vi "Process_Backup.vi"(8 "error in":errorcluster, 11 "RemoteControl":refnum<class "RemoteControl.lvclass">) -> (0 "error out":errorcluster, 3 "RemoteControl out":refnum<class "RemoteControl.lvclass">)   [LabVIEW 2016]
doc: "---------------------------------------------------------------\nJKI State Machine Objects™\nhttp://jki.net/state-machine-objects/\nCopyright (C) 2005-2015, JKI <info@jki.net>\nALL RIGHTS RESERVED"
uses:
  RemoteControl.lvclass
  <vilib>/JKI/JKI SMO/SMO/SMO.lvclass
  <vilib>/JKI/JKI SMO/SMO/Typedefs/Parent Call--Enum.ctl
  Typedefs/Message--Cluster.ctl
  Typedefs/PublicEvents--RemoteControl.SendMessageFromProcess.ctl
  <vilib>/JKI/JKI SMO/SMO/Typedefs/SMOState --Enum.ctl
  C:/user/patrick/hg/levylab_inst/lvsrc/SMOs/LevyLab/LevyLab.lvclass
  C:/Program Files (x86)/National Instruments/LabVIEW 2016/vi.lib/JKI/JKI SMO/SMO/SMO.lvclass
  Typedefs/RC Process Type--Enum.ctl
panel:
  in  "Debug Mode":bool=TRUE
  out "Servers":T1[](array[typedef])
  in  "timeout in ms (100)":i32=10
  out "Message from Server":T2 {"Message ID" format="%#_6f"}
  out "Name":string
  out "Message from Remote":T2 {"Message ID" format="%#_6f"}
  out "Message from Owner":T2 {"Message ID" format="%#_6f"}
  in  "stop":bool
  out "RC Process Type":T3
  # "For instructions on how to use the JKI State Machine Objects, examples and video tutorials, visit:\nhttp://jki.net/state-machine-objects/\n\nJKI State Machine Objects™\nhttp://jki.net/state-machine-objects/\nCopyright (C) 2005-2015, JKI <info@jki.net>\nALL RIGHTS RESERVED"
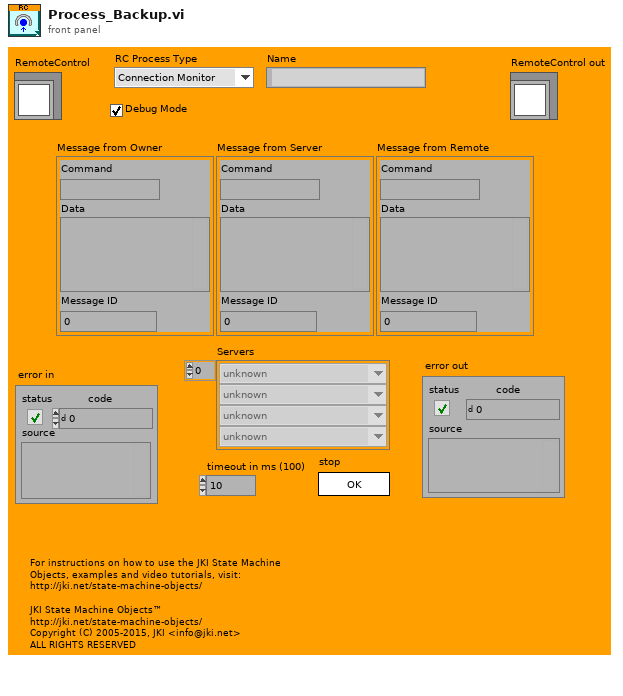
[diagram p1: front panel]
types:
  T1 = typedef "SMO.lvclass/SMOState --Enum.ctl" = enum16{"unknown", "Created", "Started", "Stopped"}
  T2 = typedef "RemoteControl.lvclass/Message--Cluster.ctl" = cluster{"Command":string, "Data":variant, "Message ID":i32}
  T3 = typedef "RemoteControl.lvclass/RC Process Type--Enum.ctl" = enum16{"Connection Monitor", "Server", "Client"}
  T4 = typedef "SMO.lvclass/Parent Call--Enum.ctl" = enum16{"Allows parent to run", "Does not request parent to run"}
  T5 = enum32{"invalid app kind", "Development System", "Run Time System", "Student Edition", "Embedded LabVIEW", "Evaluation", "Custom"}
  T6 = enum32{"Invalid", "Standard", "Closed", "Hidden", "Minimized", "Maximized"}
  T7 = enum32{"Bad", "Idle", "Run top level", "Running"}
  T8 = cluster{"Current VI Reference":refnum<vi>, "Close Panel on Exit?":bool, "error":errorcluster}
  T9 = cluster{"Core":cluster{"Current VI Reference":refnum<vi>, "Close Panel on Exit?":bool, "error":errorcluster}, "Self Reference":refnum<class "RemoteControl.lvclass">, "RC Process Type":void, "Configure":void, "Message":T2, "Servers":refnum<class "RemoteControl.lvclass">[], "Server Message":refnum<user-event>[], "Server State":refnum<user-event>[], "Server index":i32}
  T10 = typedef "SMO.lvclass/Protected Events.ctl" = cluster{"StopProcesses":refnum<user-event>, "AbortProcesses":refnum<user-event>, "Config Changed":refnum<user-event>, "Dependency":refnum<user-event>}
  T11 = typedef "RemoteControl.lvclass/PrivateEvents--Cluster.ctl" = cluster{"Configure":refnum<user-event>, "SendMessageToProcess":refnum<user-event>}
  T12 = typedef "RemoteControl.lvclass/PublicEvents--Cluster.ctl" = cluster{"SendMessageFromProcess":refnum<user-event>}
  T13 = typedef "SMO.lvclass/Public Events.ctl" = cluster{"Error":refnum<user-event>, "State":refnum<user-event>, "Reserve State":refnum<user-event>}
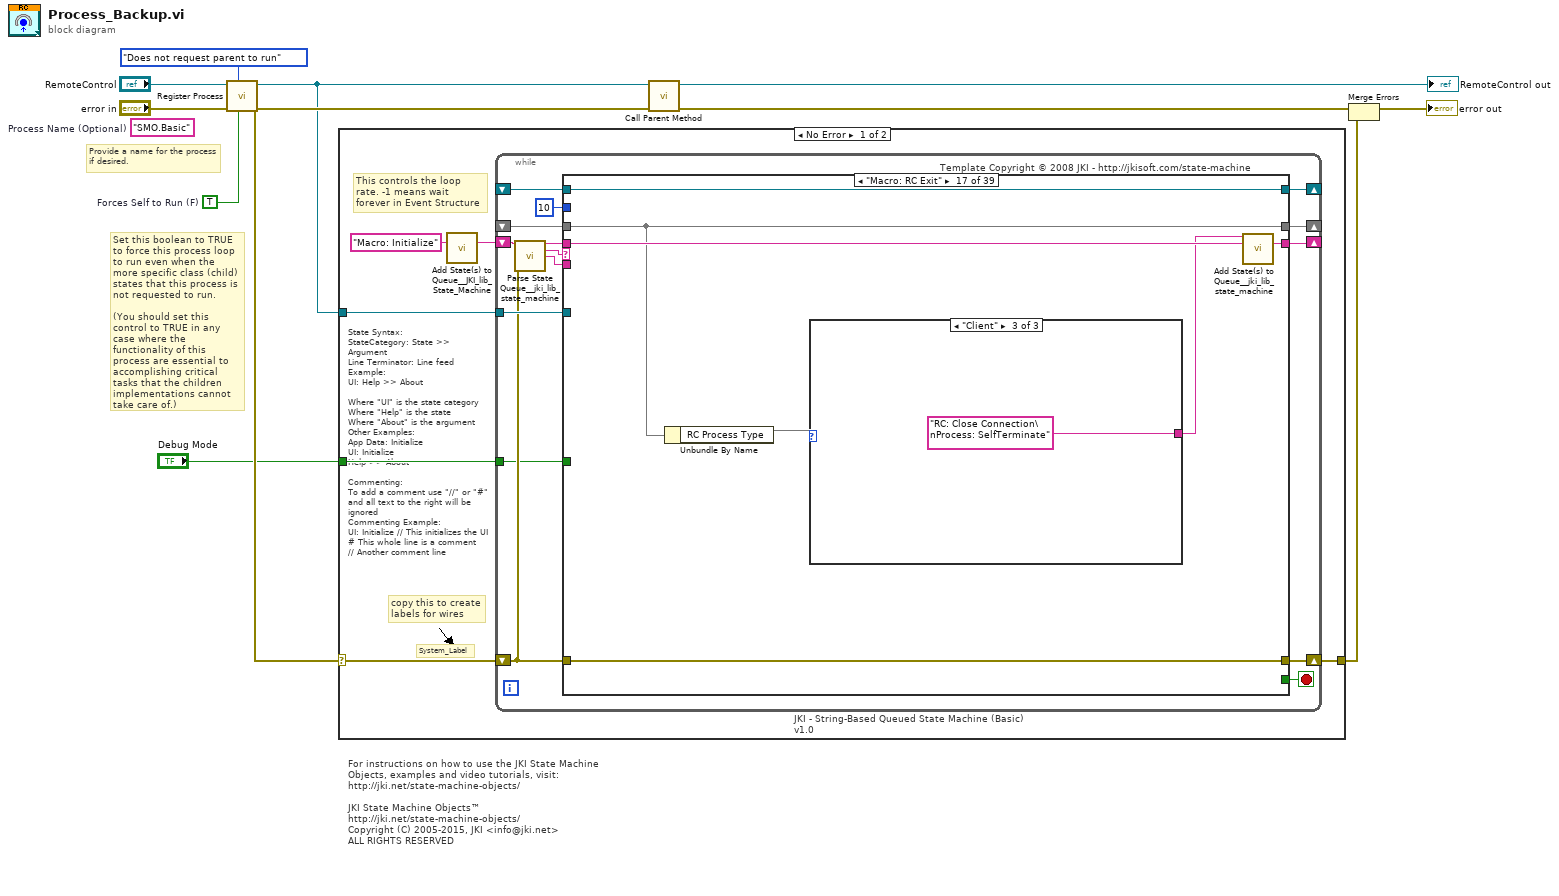
[diagram p0: block diagram]
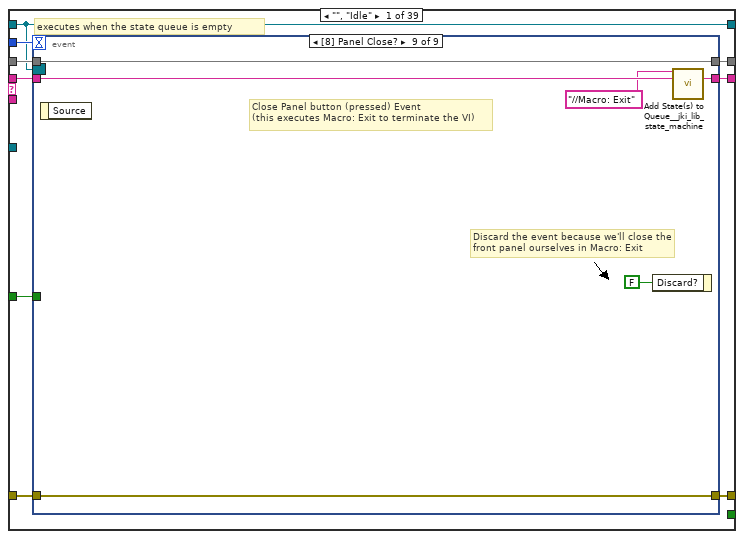
[diagram p2: hidden frame]
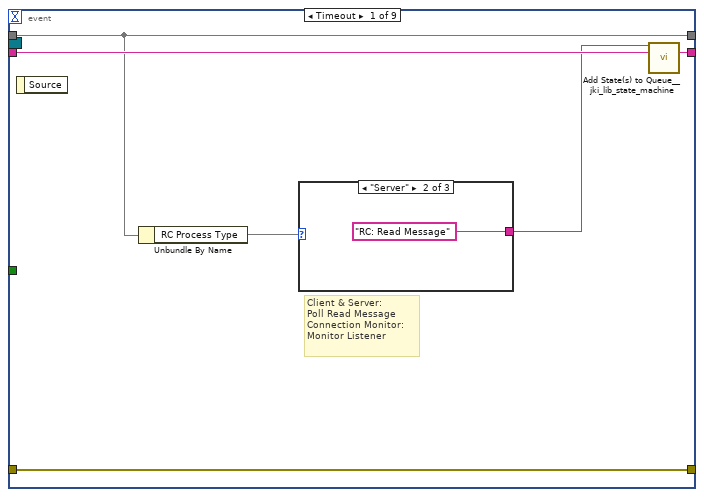
[diagram p3: hidden frame]
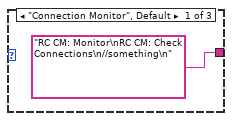
[diagram p4: hidden frame]
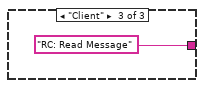
[diagram p5: hidden frame]
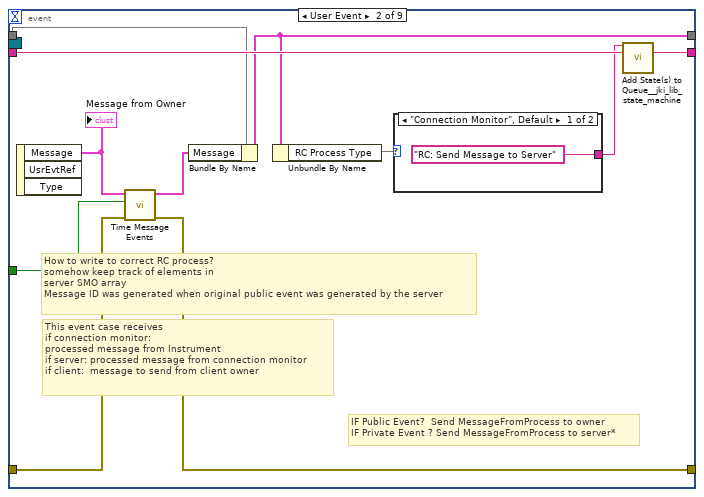
[diagram p6: hidden frame]
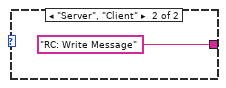
[diagram p7: hidden frame]
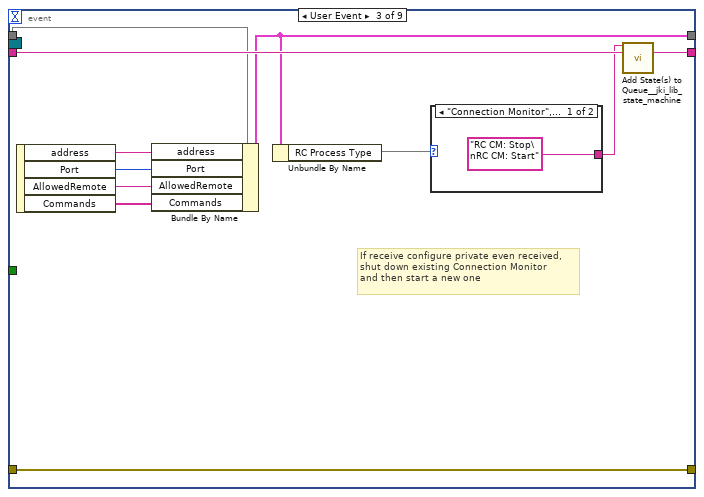
[diagram p8: hidden frame]
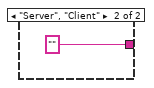
[diagram p9: hidden frame]
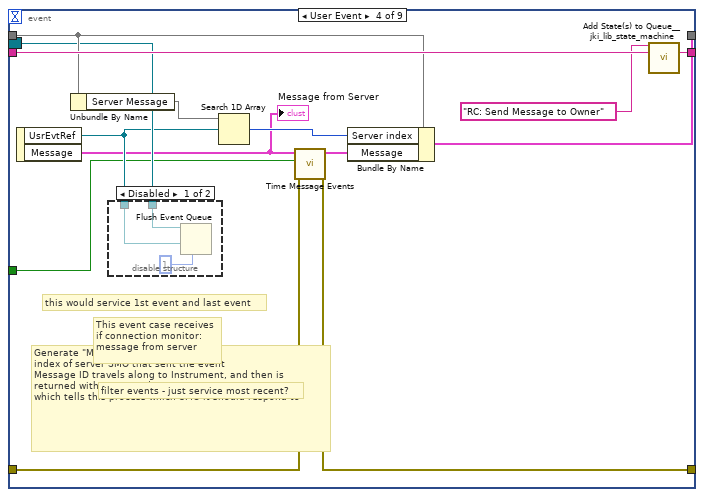
[diagram p10: hidden frame]
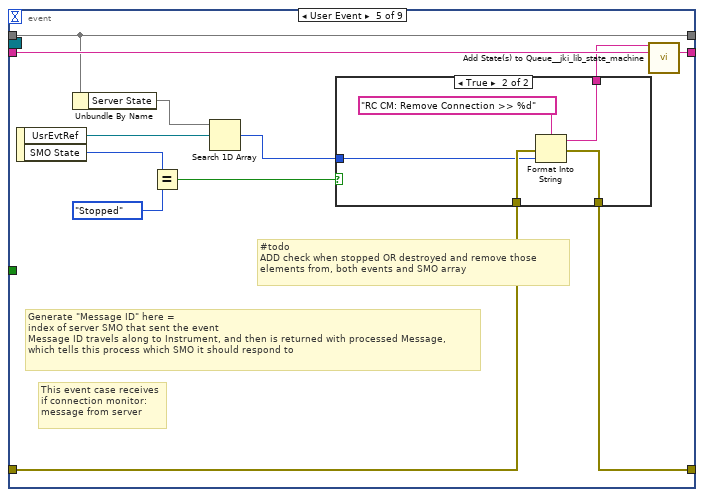
[diagram p12: hidden frame]
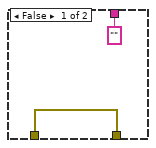
[diagram p13: hidden frame]
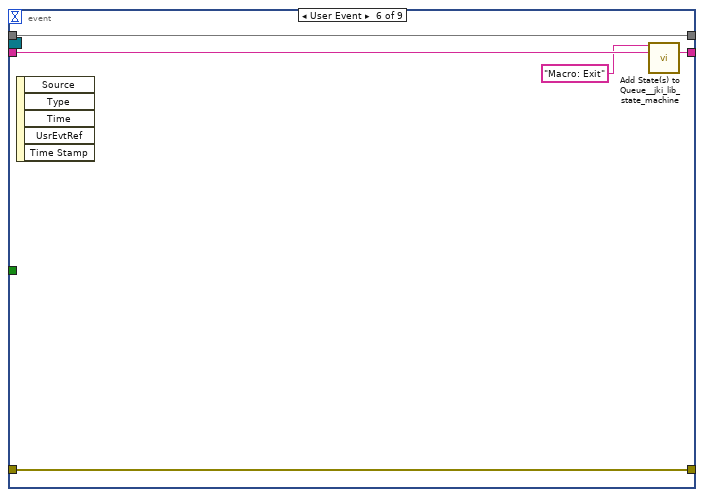
[diagram p14: hidden frame]
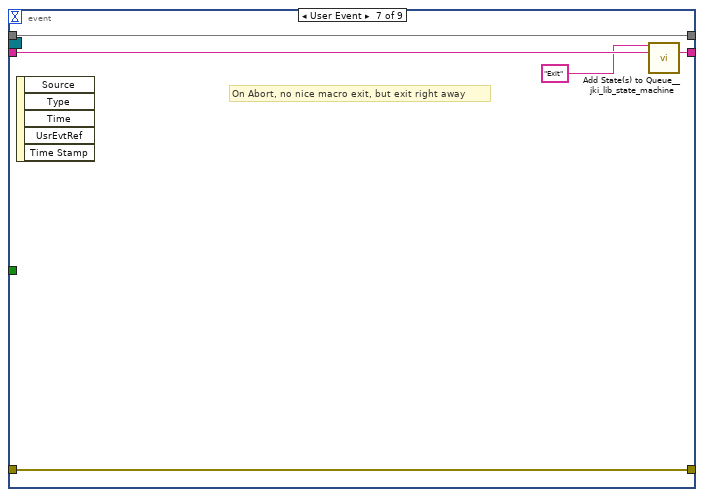
[diagram p15: hidden frame]
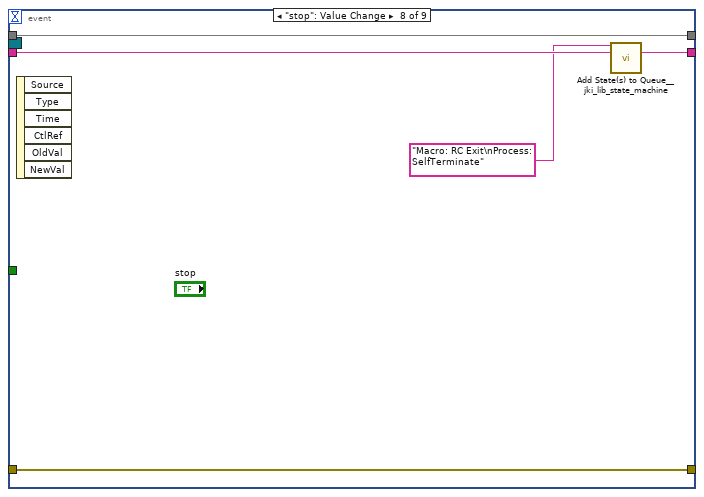
[diagram p16: hidden frame]
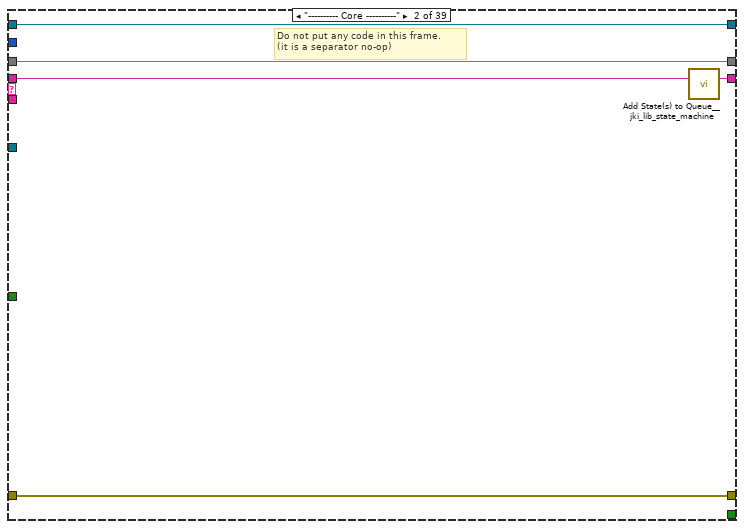
[diagram p17: hidden frame]
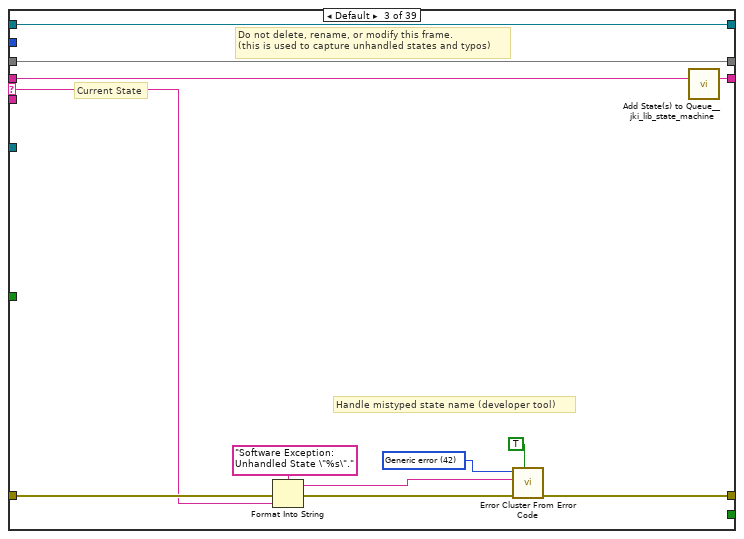
[diagram p18: hidden frame]
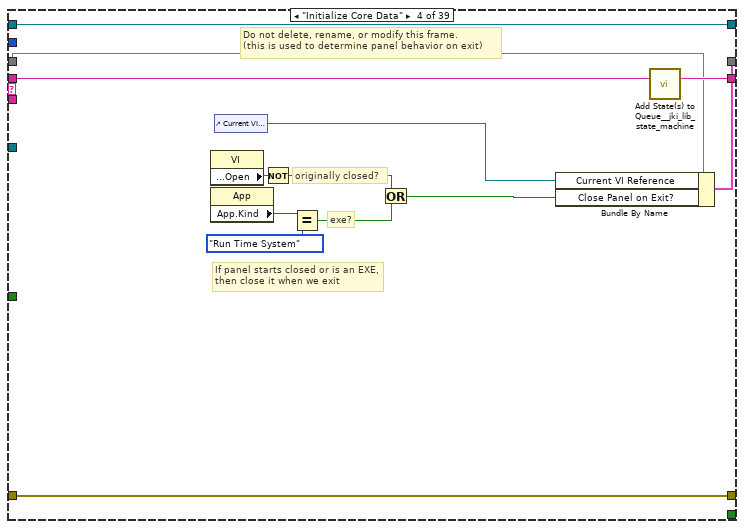
[diagram p19: hidden frame]
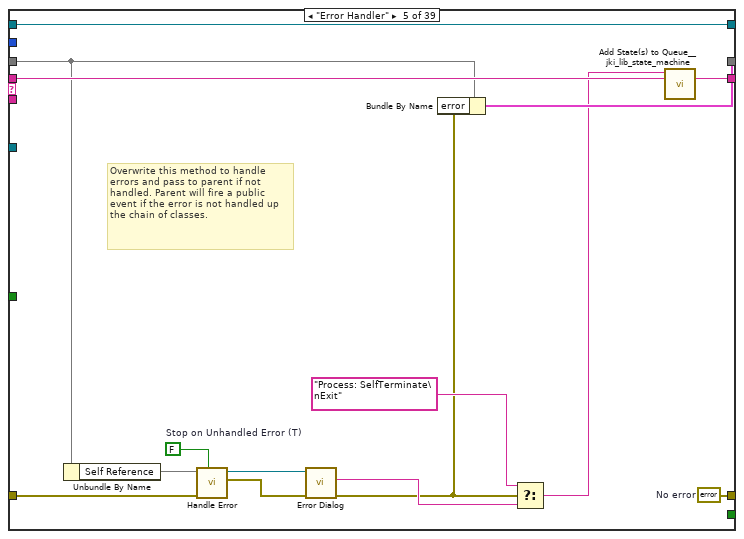
[diagram p20: hidden frame]
diagram:
  w2 = TRUE  # Forces Self to Run (F)
  (unwired) "SMO.Basic"  # Process Name (Optional)
  # "Provide a name for the process\nif desired."
  # "Set this boolean to TRUE to force this process loop to run even when the more specific class (child) states that this process is not requested to run.\n\n(You should set this control to TRUE in any case where the functionality of this process are essential to accomplishing critical tasks that the children implementations cannot take care of.)"
  # "For instructions on how to use the JKI State Machine Objects, examples and video tutorials, visit:\nhttp://jki.net/state-machine-objects/\n\nJKI State Machine Objects™\nhttp://jki.net/state-machine-objects/\nCopyright (C) 2005-2015, JKI <info@jki.net>\nALL RIGHTS RESERVED"
  n1 = call <vilib>:"Register Process.vi"("Forces Self to Run (F)"=w2, "Parent Call"=Parent_Call--Enum."Does not request parent to run", "error in (no error)"="error in", "SMO"="RemoteControl") -> ("error out"=w8:errorcluster, "SMO out"=w7:refnum<class "RemoteControl.lvclass">)  [unwired: 6 in]
  n2 = case shown="No Error" w8 {
    selector: w8 -> [w14 w602]
    tunnel: w7 -> [w15 _]
    tunnel: [w13 w602] -> w4
    tunnel: "Debug Mode" -> [w12 _]
    frame No Error {
      # "State Syntax:\nStateCategory: State >> Argument\nLine Terminator: Line feed\nExample:\nUI: Help >> About\n\nWhere \"UI\" is the state category\nWhere \"Help\" is the state\nWhere \"About\" is the argument\nOther Examples:\nApp Data: Initialize\nUI: Initialize\nHelp >> About\n\nCommenting:\nTo add a comment use \"//\" or \"#\" and all text to the right will be ignored\nCommenting Example:\nUI: Initialize // This initializes the UI\n# This whole line is a comment\n// Another comment line"
      # "copy this to create labels for wires"
      # "This controls the loop rate. -1 means wait forever in Event Structure"
      # "System_Label"
      n3 = call <vilib>:"Add State(s) to Queue__JKI_lib_State_Machine.vi"("State(s) in (\"\")"="Macro: Initialize") -> ("States Out"=w17:string)  [unwired: 14 in]
      n4 = while "JKI - String-Based Queued State Machine (Basic) v1.0" {
        shift-right: [w25] -> _
        shift-left: _ -> [w24]
        shift-right: [w28] -> w13
        shift-left: w14 -> [w19]
        shift-right: [w27] -> _
        shift-left: w17 -> [w29]
        tunnel: w15 -> [w22]
        shift-right: [w21] -> _
        shift-left: _ -> [w20]
        tunnel: w12 -> [w18]
        stop <- w26 stop-if-true
        # "Template Copyright © 2008 JKI - http://jkisoft.com/state-machine"
        n5 = call <vilib>:"Parse State Queue__jki_lib_state_machine.vi"("State Queue"=w29, "Error In (no error)"=w19) -> ("Remaining States"=w31:string, "Current State"=w32:string, "Arguments"=w30:string)  [unwired: 11 in]
        n6 = case shown="\"Macro: RC Exit\"" w32 {
          selector: w32 -> [_ _ w140 _ _ _ _ _ _ _ _ _ _ _ _ _ _ _ _ _ _ _ _ _ _ _ _ _ _ _ _ _ _ _ _ _ _ _ _]
          tunnel: w31 -> [w41 w138 w144 w163 w178 w184 w189 w206 w213 w218 w233 w244 w262 w292 w306 w315 w325 w342 w347 w358 w367 w372 w387 w393 w398 w410 w424 w440 w469 w478 w487 w496 w501 w511 w525 w544 w579 w594 w601]
          tunnel: w30 -> [_ _ _ _ _ _ _ _ _ _ _ w238 w257 _ _ _ _ _ _ _ _ _ _ _ _ _ _ _ _ _ _ _ _ _ _ _ w573 w590 _]
          tunnel: w24 -> [w39 w135 w142 w154 w174 w180 w186 _ w209 w215 w230 w242 w259 w289 w302 w310 w319 w334 w344 w355 w363 w369 w385 w391 w396 w407 w421 w427 w464 w470 w480 w491 w499 w503 w515 w541 w571 w592 w598]
          tunnel: [w38 w136 w146 w160 w175 w179 w187 w203 w210 w216 w226 w239 w253 w290 w304 w308 w323 w340 w345 w350 w359 w370 w381 w389 w394 w406 w420 w428 w465 w474 w482 w488 w497 w508 w519 w539 w577 w589 w595] -> w28
          tunnel: w19 -> [w37 w136 w145 w160 w166 _ w187 w204 w211 w216 w227 w240 w260 w290 w304 w309 w323 w340 w345 w351 w360 w370 w382 w389 w394 w401 w415 w437 w461 w475 w483 w493 w497 w509 w517 w540 w564 w589 w596]
          tunnel: [w40 w137 w143 w162 w177 w183 w188 w205 w212 w217 w232 w243 w261 w291 w305 w314 w324 w341 w346 w357 w366 w371 w386 w392 w397 w409 w423 w439 w468 w477 w486 w495 w500 w510 w524 w543 w578 w593 w600] -> w27
          tunnel: [_ _ _ _ _ TRUE _ _ _ _ _ _ _ _ _ _ _ _ _ _ _ _ _ _ _ _ _ _ _ _ _ _ _ _ _ _ _ _ _] -> w26
          tunnel: [w36 w135 w142 w161 w173 w180 w186 w198 w209 w215 w230 w242 w259 w289 w302 w310 w319 w334 w344 w355 w364 w369 w385 w391 w396 w407 w421 w426 w464 w471 w479 w490 w499 w502 w514 w541 w570 w591 w598] -> w25
          tunnel: 10 ("Timeout") -> [w35 _ _ _ _ _ _ _ _ _ _ _ _ _ _ _ _ _ _ _ _ _ _ _ _ _ _ _ _ _ _ _ _ _ _ _ _ _ _]
          tunnel: w22 -> [_ _ _ _ _ _ _ w201 _ _ _ _ _ _ _ _ _ _ _ _ _ _ _ _ _ _ _ _ _ _ _ _ _ _ _ _ _ _ _]
          tunnel: [w34 w134 w139 w151 w176 w181 w185 w200 w208 w214 w231 w241 w256 w288 w303 w313 w322 w335 w343 w356 w365 w368 w384 w390 w395 w408 w422 w438 w467 w476 w485 w494 w498 w505 w520 w542 w568 w587 w599] -> w21
          tunnel: w20 -> [w34 w134 w139 w151 w176 w181 w185 w200 w208 w214 w231 w241 w256 w288 w303 w313 w322 w335 w343 w356 w365 w368 _ w390 w395 w408 w422 w438 w467 w476 w485 w494 w498 w505 w520 w542 w569 w588 w599]
          tunnel: w18 -> [w33 _ _ _ _ _ _ _ _ _ _ _ _ _ _ _ _ _ _ _ _ _ _ _ _ w402 w418 w425 w463 _ _ _ _ _ _ _ _ _ _]
          frame "", "Idle" {
            # "executes when the state queue is empty"
            n7 = event shown="[8] Panel Close?" {
              selector: w34 -> [_ _ _ w85 _ _ _ _ _]
              dyn-events: _ -> [_ _ _ _ _ _ _ _ _]
              timeout: w35 -> [_ _ _ _ _ _ _ _ _]
              tunnel: w41 -> [w47 w61 w73 w90 w105 w117 w122 w126 w133]
              tunnel: [w46 w60 w72 w89 w104 w116 w121 w127 w132] -> w40
              tunnel: w39 -> [w42 w59 w71 w88 w101 w114 w119 w125 w130]
              tunnel: [w45 w52 w74 w81 w97 w115 w120 w123 w131] -> w38
              tunnel: w37 -> [w45 w53 w74 w82 w98 w115 w120 w123 w131]
              tunnel: [w42 w57 w69 w87 w101 w114 w119 w125 w130] -> w36
              tunnel: w33 -> [_ w51 _ w77 _ _ _ _ _]
              event Timeout {
                # "Client & Server:\nPoll Read Message\nConnection Monitor:\nMonitor Listener"
                n8 = event-data() -> ()  [unwired: 1 in, 1 out]
                n9 = Unbundle By Name(w42) -> ("RC Process Type"=w44)
                n10 = case shown="\"Server\"" w44 {
                  tunnel: ["RC CM: Monitor\nRC CM: Check Connections\n//something\n" ("State(s) in Front (\"\")") "RC: Read Message" ("State(s) in Front (\"\")") "RC: Read Message" ("State(s) in Front (\"\")")] -> w43
                  frame "Connection Monitor", Default {
                  }
                  frame "Server" {
                  }
                  frame "Client" {
                  }
                }
                n11 = call <vilib>:"Add State(s) to Queue__jki_lib_state_machine.vi"("State(s) in Front (\"\")"=w43, "State(s) in (\"\")"=w47) -> ("States Out"=w46:string)  [unwired: 13 in]
              }
              event User Event {
                # "IF Public Event?  Send MessageFromProcess to owner\nIF Private Event ? Send MessageFromProcess to server*"
                # "How to write to correct RC process?\nsomehow keep track of elements in\nserver SMO array\nMessage ID was generated when original public event was generated by the server"
                # "This event case receives\nif connection monitor:\nprocessed message from Instrument\nif server: processed message from connection monitor\nif client:  message to send from client owner"
                n12 = event-data() -> ("Message"=w55:T2)  [unwired: 1 in, 2 out]
                "Message from Owner" <- w55
                n13 = call "Time Message Events.vi"("error in (no error)"=w53, "Debug Mode"=w51, "Message in"=w55) -> ("error out"=w52:errorcluster, "Message out"=w54:T2)  [unwired: 6 in, 1 out]
                n14 = Bundle By Name(cluster=w59, "Message"=w54) -> (w57:cluster{})
                n15 = Unbundle By Name(w57) -> ("RC Process Type"=w58)
                n16 = case shown="\"Connection Monitor\", Default" w58 {
                  tunnel: ["RC: Send Message to Server" ("State(s) in Front (\"\")") "RC: Write Message" ("State(s) in Front (\"\")")] -> w56
                  frame "Connection Monitor", Default {
                  }
                  frame "Server", "Client" {
                  }
                }
                n17 = call <vilib>:"Add State(s) to Queue__jki_lib_state_machine.vi"("State(s) in Front (\"\")"=w56, "State(s) in (\"\")"=w61) -> ("States Out"=w60:string)  [unwired: 13 in]
              }
              event User Event {
                # "If receive configure private even received,\nshut down existing Connection Monitor \nand then start a new one"
                n18 = event-data() -> ("address"=w64:string, "Port"=w65:u16, "AllowedRemote"=w66:string, "Commands"=w67:string[])  [unwired: 1 in]
                n19 = Bundle By Name(cluster=w71, "address"=w64, "Port"=w65, "AllowedRemote"=w66, "Commands"=w67) -> (w69:cluster{})
                n20 = Unbundle By Name(w69) -> ("RC Process Type"=w70)
                n21 = case shown="\"Connection Monitor\", Default" w70 {
                  tunnel: ["RC CM: Stop\nRC CM: Start" ("State(s) in Front (\"\")") "" ("State(s) in Front (\"\")")] -> w68
                  frame "Connection Monitor", Default {
                  }
                  frame "Server", "Client" {
                  }
                }
                n22 = call <vilib>:"Add State(s) to Queue__jki_lib_state_machine.vi"("State(s) in Front (\"\")"=w68, "State(s) in (\"\")"=w73) -> ("States Out"=w72:string)  [unwired: 13 in]
              }
              event User Event {
                # "this would service 1st event and last event"
                # "filter events - just service most recent?"
                # "This event case receives\nif connection monitor:\nmessage from server"
                # "Generate \"Message ID\" here = \nindex of server SMO that sent the event\nMessage ID travels along to Instrument, and then is returned with processed Message,\nwhich tells this process which SMO it should respond to"
                n23 = event-data() -> ("UsrEvtRef"=w84:refnum<user-event>, "Message"=w79:T2)  [unwired: 1 in]
                "Message from Server" <- w79
                n24 = Unbundle By Name(w88) -> ("Server Message"=w86)
                n25 = disable-structure shown="Disabled" {
                  disable-tunnel: w85 -> [w93 _]
                  disable-tunnel: w84 -> [w92 _]
                  frame Disabled {
                    n26 = Flush Event Queue(0:w93, 2:w92, 5:1 ("keep most recent")) -> ()  [unwired: 3 in, 3 out]
                  }
                  frame Enabled {
                  }
                }
                n27 = Search 1D Array(1D array=w86, element=w84) -> (index of element=w80:i32)  [unwired: 1 in]
                n28 = call "Time Message Events.vi"("error in (no error)"=w82, "Debug Mode"=w77, "Message in"=w79) -> ("error out"=w81:errorcluster, "Message out"=w83:T2)  [unwired: 6 in, 1 out]
                n29 = Bundle By Name(cluster=w88, "Server index"=w80, "Message"=w83) -> (w87:cluster{})
                n30 = call <vilib>:"Add State(s) to Queue__jki_lib_state_machine.vi"("State(s) in Front (\"\")"="RC: Send Message to Owner", "State(s) in (\"\")"=w90) -> ("States Out"=w89:string)  [unwired: 13 in]
              }
              event User Event {
                # "#todo\nADD check when stopped OR destroyed and remove those\nelements from, both events and SMO array"
                # "This event case receives\nif connection monitor:\nmessage from server"
                # "Generate \"Message ID\" here = \nindex of server SMO that sent the event\nMessage ID travels along to Instrument, and then is returned with processed Message,\nwhich tells this process which SMO it should respond to"
                n31 = event-data() -> ("UsrEvtRef"=w103:refnum<user-event>, "SMO State"=w94:T1)  [unwired: 1 in]
                n32 = Unbundle By Name(w101) -> ("Server State"=w102)
                n33 = Equal?(x=w94, y=SMOState_--Enum."Stopped" ("SMO State")) -> (x = y?=w95:bool)
                n34 = Search 1D Array(1D array=w102, element=w103) -> (index of element=w96:i32)  [unwired: 1 in]
                n35 = case shown="True" w95 {
                  tunnel: ["" w111] -> w99
                  tunnel: w98 -> [w106 w110]
                  tunnel: [w106 w109] -> w97
                  tunnel: w96 -> [_ w108]
                  frame False {
                  }
                  frame True {
                    n36 = Format Into String(format string="RC CM: Remove Connection >> %d", error in=w110, w108) -> (resulting string=w111:string, error out=w109:errorcluster)  [unwired: 1 in]
                  }
                }
                n37 = call <vilib>:"Add State(s) to Queue__jki_lib_state_machine.vi"("State(s) in Front (\"\")"=w99, "State(s) in (\"\")"=w105) -> ("States Out"=w104:string)  [unwired: 13 in]
              }
              event User Event {
                n38 = event-data() -> ()  [unwired: 1 in, 5 out]
                n39 = call <vilib>:"Add State(s) to Queue__jki_lib_state_machine.vi"("State(s) in Front (\"\")"="Macro: Exit", "State(s) in (\"\")"=w117) -> ("States Out"=w116:string)  [unwired: 13 in]
              }
              event User Event {
                # "On Abort, no nice macro exit, but exit right away"
                n40 = event-data() -> ()  [unwired: 1 in, 5 out]
                n41 = call <vilib>:"Add State(s) to Queue__jki_lib_state_machine.vi"("State(s) in Front (\"\")"="Exit", "State(s) in (\"\")"=w122) -> ("States Out"=w121:string)  [unwired: 13 in]
              }
              event "stop": Value Change {
                n42 = event-data() -> ()  [unwired: 1 in, 6 out]
                n43 = call <vilib>:"Add State(s) to Queue__jki_lib_state_machine.vi"("State(s) in Front (\"\")"="Macro: RC Exit\nProcess: SelfTerminate" ("State(s) in Front (\"\")"), "State(s) in (\"\")"=w126) -> ("States Out"=w127:string)  [unwired: 13 in]
              }
              event Panel Close? {
                # "Discard the event because we'll close the front panel ourselves in Macro: Exit"
                # "Close Panel button (pressed) Event\n(this executes Macro: Exit to terminate the VI)"
                n44 = event-data() -> ()  [unwired: 1 in, 1 out]
                n45 = event-data("Discard?"=FALSE) -> ()  [unwired: 1 in, 1 out]
                n46 = call <vilib>:"Add State(s) to Queue__jki_lib_state_machine.vi"("State(s) in Front (\"\")"="//Macro: Exit", "State(s) in (\"\")"=w133) -> ("States Out"=w132:string)  [unwired: 13 in]
              }
            }
          }
          frame "---------- Core ----------" {
            # "Do not put any code in this frame.\n(it is a separator no-op)"
            n47 = call <vilib>:"Add State(s) to Queue__jki_lib_state_machine.vi"("State(s) in (\"\")"=w138) -> ("States Out"=w137:string)  [unwired: 14 in]
          }
          frame Default {
            w149 = 42 items=["No error", "Argument error", "Memory is full", "Out of zone", "End of file", "File already open", "Generic file I/O error", "File not found", "File permission error", "Disk is full", "Duplicate path", "Too many files open", "System feature not enabled", "Resource file not found", "Cannot add resource", "Resource not found", "Image not found", "Image memory error", "Pen does not exist", "Config type invalid", "Config token not found", "Config parse error", "Config memory error", "Bad external code format", "Bad external code offset", "External code not present", "Null window", "Destroy window error", "Null menu", "Print aborted", "Bad print record", "Print driver error", "Windows error during printing", "Memory error during printing", "Print dialog error", "Generic print error", "Invalid device refnum", "Device not found", "Device parameter error", "Device unit error", "Cannot open device", "Device call aborted", "Generic error", "Cancelled by user", "Object ID too low", "Object ID too high", "Object not in heap", "Unknown heap", "Unknown object (invalid DefProc)", "Unknown object (DefProc not in table)", "Message out of range", "Invalid (null) method", "Unknown message", "Manager call not supported", "Bad address", "Network operation in progress", "Network operation timed out", "Connection is busy", "Network attribute not supported", "Network error", "Address in use", "System out of memory", "Connection aborted", "Connection refused", "Not connected", "Already connected", "Connection closed", "Initialization error (interapplication manager)", "Bad occurrence", "Wait on unbound occurrence handler", "Occurrence queue overflow", "Datalog type conflict", "Unused", "Unrecognized type (interapplication manager)", "Memory corrupt", "Failed to make temporary DLL", "Old CIN version", "Drag socket not found", "Failed to load drop-object", "Failed to register OLE object", "Failed to release OLE object", "Format specifier type mismatch", "Unknown format specifier", "Too few format specifiers", "Too many format specifiers", "Scan failed", "Newer CIN version", "Error converting to variant", "Runtime menu error", "Password tampered", "Variant attribute not found", "Incompatible variant data type", "Event data is not available", "Event Store is not present", "Occurrence is not found", "Event Queue is not created", "Event info is not available", "Refnum passed is NULL", "Error retrieving Class GUID", "Error retrieving CoClass GUID", "Error retrieving TypeLib GUID.", "Bad built application magic bytes.", "Specific driver is different from the specific driver associated with the Logical Name.", "There is no session opened to the class driver.", "Max Error", "MAX - Error with config objects", "MAX - Error loading configuration", "MAX - Group not supported"]
            # "Current State"
            # "Do not delete, rename, or modify this frame.\n(this is used to capture unhandled states and typos)"
            # "Handle mistyped state name (developer tool)"
            n48 = Format Into String(format string="Software Exception: Unhandled State \"%s\"." ("message"), error in=w145, w140) -> (resulting string=w148:string, error out=w147:errorcluster)  [unwired: 1 in]
            n49 = call <vilib>:"Error Cluster From Error Code.vi"("show call chain? (False)"=TRUE, "error in (no error)"=w147, "error message (\"\")"=w148, "error code (0)"=w149) -> ("error out"=w146:errorcluster)  [unwired: 5 in]
            n50 = call <vilib>:"Add State(s) to Queue__jki_lib_state_machine.vi"("State(s) in (\"\")"=w144) -> ("States Out"=w143:string)  [unwired: 14 in]
          }
          frame "Initialize Core Data" {
            # "Do not delete, rename, or modify this frame.\n(this is used to determine panel behavior on exit)"
            # "originally closed?"
            # "exe?"
            # "If panel starts closed or is an EXE, then close it when we exit"
            n51 = property class="VI"() -> ("Front Panel.Open"=w159:bool)  [unwired: 2 in, 2 out]
            n52 = property class="App"() -> ("App.Kind"=w158:T5)  [unwired: 2 in, 2 out]
            n53 = control-ref of="Current VI Reference"() -> (w152:refnum<vi>)
            n54 = Not(x=w159) -> (.not. x?=w156:bool)
            n55 = Equal?(x=w158, y=T5."Run Time System" ("Application:Kind")) -> (x = y?=w155:bool)
            n56 = Or(x=w156, y=w155) -> (x .or. y?=w153:bool)
            n57 = Bundle By Name(cluster=w154, "Current VI Reference"=w152, "Close Panel on Exit?"=w153) -> (w161:cluster{})
            n58 = call <vilib>:"Add State(s) to Queue__jki_lib_state_machine.vi"("State(s) in (\"\")"=w163) -> ("States Out"=w162:string)  [unwired: 14 in]
          }
          frame "Error Handler" {
            w171 = FALSE  # Stop on Unhandled Error (T)
            w175 = errorcluster {"status"=FALSE, "code"=0, "source"=""}  # No error
            # "Overwrite this method to handle errors and pass to parent if not handled. Parent will fire a public event if the error is not handled up the chain of classes."
            n59 = Unbundle By Name(w174) -> ("Self Reference"=w170)
            n60 = call-dynamic "Handle Error.vi"("Stop on Unhandled Error (T)"=w171, "error in"=w166, "LevyLab"=w170) -> ("Unhandled error"=w164:errorcluster, "LevyLab out"=w167:refnum<class "RemoteControl.lvclass">)  [unwired: 6 in, 1 out]
            n61 = call "Error Dialog.vi"("error in (no error)"=w164, "RemoteControl in"=w167) -> ("error out"=w165:errorcluster, "States to Execute"=w168:string)  [unwired: 7 in, 1 out]
            n62 = Bundle By Name(cluster=w174, "error"=w165) -> (w173:cluster{})
            n63 = Select(t="Process: SelfTerminate\nExit", s=w165, f=w168) -> (s? t:f=w169:string)
            n64 = call <vilib>:"Add State(s) to Queue__jki_lib_state_machine.vi"("State(s) in Front (\"\")"=w169, "State(s) in (\"\")"=w178) -> ("States Out"=w177:string)  [unwired: 13 in]
          }
          frame "Exit" {
            # "Do not put any code in this frame.\n(No errors that occur here will be handled.)"
            n65 = Unbundle By Name(w180) -> ("Core.error"=w179)
            n66 = call <vilib>:"Add State(s) to Queue__jki_lib_state_machine.vi"("State(s) in (\"\")"=w184) -> ("States Out"=w183:string)  [unwired: 14 in]
          }
          frame "---------- Data ----------" {
            # "Do not put any code in this frame.\n(It is a separator no-op. You can make a copy of this frame to create a new Data frame)"
            n67 = call <vilib>:"Add State(s) to Queue__jki_lib_state_machine.vi"("State(s) in (\"\")"=w189) -> ("States Out"=w188:string)  [unwired: 14 in]
          }
          frame "Data: Initialize" {
            w193 = 0  # Server index
            w192 = refnum<user-event>[] [] items=["unknown", "Created", "Started", "Stopped"]  # Server State
            w191 = refnum<user-event>[] []  # Server Message
            w190 = refnum<class "RemoteControl.lvclass">[] []  # Servers
            w197 = T2 {"Command"="", "Data"=variant, "Message ID"=0}  # Message
            w199 = T8 {"Current VI Reference"=refnum, "Close Panel on Exit?"=FALSE, "error"={"status"=FALSE, "code"=0, "source"=""}}  # Core
            w202 = refnum<class "RemoteControl.lvclass"> refnum  # Self Reference
            # "#todo\nwould these be better as array of cluster?"
            # "do not delete - used by framework"
            # "Data names and types of shift register data are defined by this bundle."
            # "Initialize the shift-register data, here.\n(data names are defined by what you wire into the bundle function)"
            n68 = Variant To Data(error in=w204, type=w202, Variant=w201) -> (data=w196:refnum<class "RemoteControl.lvclass">, error out=w203:errorcluster)
            n69 = Unbundle By Name(w196) -> ("RC Process Type"=w194, "Configure"=w195)
            n70 = Bundle("Core"=w199, "Self Reference"=w196, "RC Process Type"=w194, "Configure"=w195, "Message"=w197, "Servers"=w190, "Server Message"=w191, "Server State"=w192, "Server index"=w193) -> (w198:T9)  [unwired: 1 in]
            n71 = call <vilib>:"Add State(s) to Queue__jki_lib_state_machine.vi"("State(s) in (\"\")"=w206) -> ("States Out"=w205:string)  [unwired: 14 in]
          }
          frame "Data: Cleanup" {
            # "Cleanup any data and references, here.\n(this is called automatically, by the Macro: Exit)"
            n72 = Unbundle By Name(w209) -> ("Core.Current VI Reference"=w207)
            n73 = Close Reference(reference=w207, error in (no error)=w211) -> (error out=w210:errorcluster)
            n74 = call <vilib>:"Add State(s) to Queue__jki_lib_state_machine.vi"("State(s) in (\"\")"=w213) -> ("States Out"=w212:string)  [unwired: 14 in]
          }
          frame "---------- UI ----------" {
            # "Do not put any code in this frame.\n(It is a separator no-op. You can make a copy of this frame to create a new UI frame)"
            n75 = call <vilib>:"Add State(s) to Queue__jki_lib_state_machine.vi"("State(s) in (\"\")"=w218) -> ("States Out"=w217:string)  [unwired: 14 in]
          }
          frame "UI: Initialize" {
            # "Initialize the User Interface, here.\n(this is called automatically, by the Macro: Init)"
            n76 = Unbundle By Name(w230) -> ("Self Reference"=w229, "RC Process Type"=w223)
            n77 = call <vilib>:"GetName.vi"("error in (no error)"=w227, "SMO"=w229) -> ("error out"=w226:errorcluster, "Name"=→"Name":string)  [unwired: 6 in, 2 out]
            n78 = control-ref of="Message from Remote"() -> (w221:refnum<vi>)
            n79 = control-ref of="Message from Server"() -> (w219:refnum<vi>)
            n80 = case shown="\"Connection Monitor\", Default" w223 {
              tunnel: [w234 w237] -> w222
              tunnel: w221 -> [w235 w237]
              tunnel: [w235 w236] -> w220
              tunnel: w219 -> [w234 w236]
              frame "Connection Monitor", Default {
              }
              frame "Server" {
              }
            }
            n81 = property class="Clust (strict)"(reference=w220, "Visible"=FALSE) -> ()  [unwired: 1 in, 2 out]
            n82 = property class="Clust (strict)"(reference=w222, "Visible"=TRUE) -> ()  [unwired: 1 in, 2 out]
            n83 = call <vilib>:"Add State(s) to Queue__jki_lib_state_machine.vi"("State(s) in (\"\")"=w233) -> ("States Out"=w232:string)  [unwired: 14 in]
          }
          frame "UI: Cursor Set" {
            # "Argument"
            # "Initialize the User Interface, here.\n(this is called automatically, by the Macro: Init)"
            n84 = disable-structure shown="Default" {
              disable-tunnel: w240 -> [w245 w248]
              disable-tunnel: [w245 w247] -> w239
              disable-tunnel: w238 -> [_ w246]
              frame condition #0 {
              }
              frame condition #1 (active) {
                n85 = case shown="\"Idle\", Default" w246 {
                  tunnel: w248 -> [w250 w252]
                  tunnel: [w249 w251] -> w247
                  frame "Idle", Default {
                    n86 = call <vilib>:"Unset Busy.vi"("error in (no error)"=w250) -> ("error out"=w249:errorcluster)  [unwired: 10 in]
                  }
                  frame "Busy" {
                    n87 = call <vilib>:"Set Busy.vi"("error in (no error)"=w252) -> ("error out"=w251:errorcluster)  [unwired: 9 in, 1 out]
                  }
                }
              }
            }
            n88 = call <vilib>:"Add State(s) to Queue__jki_lib_state_machine.vi"("State(s) in (\"\")"=w244) -> ("States Out"=w243:string)  [unwired: 14 in]
          }
          frame "UI: Front Panel State" {
            # "Argument"
            # "Set Front Panel Open or Closed\n(Usage: \"UI: Front Panel State >> Open|Close\")"
            n89 = Unbundle By Name(w259) -> ("Core.Current VI Reference"=w258)
            n90 = disable-structure shown="Default" {
              disable-tunnel: w260 -> [w266 w287]
              disable-tunnel: [w265 w287] -> w254
              disable-tunnel: w258 -> [w264 _]
              disable-tunnel: w257 -> [w263 _]
              frame condition #0 (active) {
                n91 = case shown="\"Close\"" w263 {
                  tunnel: w266 -> [w270 w281]
                  tunnel: [w271 w282] -> w265
                  tunnel: w264 -> [_ _]
                  frame "Open", Default {
                    n92 = property class="VI"(error in=w270) -> (reference out=w268:refnum<vi>, error out=w269:errorcluster, "FP.State"=w267:T6)  [unwired: 1 in]
                    n93 = case shown="\"Closed\"" w267 {
                      tunnel: [w274 w277] -> w271
                      tunnel: w269 -> [w273 w277]
                      tunnel: w268 -> [w272 _]
                      frame "Closed" {
                        n94 = invoke class="VI" method="FP.Open"(reference=w272, error in=w273, "Activate"=TRUE, "State"=T6."Standard") -> (error out=w274:errorcluster)  [unwired: 1 in, 4 out]
                      }
                      frame Default {
                      }
                    }
                  }
                  frame "Close" {
                    n95 = property class="VI"(error in=w281) -> (reference out=w279:refnum<vi>, error out=w280:errorcluster, "FP.State"=w278:T6)  [unwired: 1 in]
                    n96 = case shown="Default" w278 {
                      tunnel: [w283 w286] -> w282
                      tunnel: w280 -> [w283 w285]
                      tunnel: w279 -> [_ w284]
                      frame "Invalid", "Closed" {
                      }
                      frame Default {
                        n97 = invoke class="VI" method="FP.Close"(reference=w284, error in=w285) -> (error out=w286:errorcluster)  [unwired: 1 in, 2 out]
                      }
                    }
                  }
                }
              }
              frame condition #1 {
              }
            }
            n98 = call <userlib>:"Wait (ms)__ogtk.vi"("error in (no error)"=w254, "milliseconds to wait"=u32 0) -> ("error out"=w253:errorcluster)  [unwired: 8 in, 1 out]
            n99 = call <vilib>:"Add State(s) to Queue__jki_lib_state_machine.vi"("State(s) in (\"\")"=w262) -> ("States Out"=w261:string)  [unwired: 14 in]
          }
          frame "---------- Macro ----------" {
            # "Do not put any code in this frame.\n(It is a separator no-op. You can make a copy of this frame to create a new Macro frame)"
            n100 = call <vilib>:"Add State(s) to Queue__jki_lib_state_machine.vi"("State(s) in (\"\")"=w292) -> ("States Out"=w291:string)  [unwired: 14 in]
          }
          frame "Macro: Initialize" {
            w297 = "UI: Initialize\nUI: Front Panel State >> Open\nMacro: RC Initialize"  # UI: Initialize UI: Front Panel State >> Open Macro: RC Initialize
            w293 = "Process: Sync"
            # "Initialization Macro\n(This is called once, when the VI starts)"
            n101 = control-ref of="This VI"() -> (w295:refnum<vi>)
            n102 = property class="VI"(reference=w295) -> ("Exec.State"=w294:T7)  [unwired: 1 in, 2 out]
            n103 = Equal?(x=w294, y=T7."Run top level") -> (x = y?=w300:bool)
            n104 = Select(t=w293, s=w300, f="") -> ()  [unwired: 1 out]
            n105 = call <vilib>:"Add State(s) to Queue__jki_lib_state_machine.vi"("State(s) in Front (\"\")"="Data: Initialize\nInitialize Core Data\nEvents: Register", "State(s) in (\"\")"=w293, "State(s) at Back (\"\")"=w297) -> ("States Out"=w296:string)  [unwired: 12 in]
            n106 = call <vilib>:"Add State(s) to Queue__jki_lib_state_machine.vi"("State(s) in Front (\"\")"=w296, "State(s) in (\"\")"=w306) -> ("States Out"=w305:string)  [unwired: 13 in]
          }
          frame "Macro: RC Initialize" {
            n107 = Unbundle By Name(w310) -> ("RC Process Type"=w312)
            "RC Process Type" <- w312
            n108 = case shown="\"Server\"" w312 {
              tunnel: ["RC CM: Start" ("State(s) in Front (\"\")") "RC: Open Server Connection" ("State(s) in Front (\"\")") "RC: Open Client Connection" ("State(s) in Front (\"\")")] -> w311
              frame "Connection Monitor", Default {
              }
              frame "Server" {
              }
              frame "Client" {
              }
            }
            n109 = call <userlib>:"Wait (ms)__ogtk.vi"("error in (no error)"=w309, "milliseconds to wait"=u32 0) -> ("error out"=w308:errorcluster)  [unwired: 8 in, 1 out]
            n110 = call <vilib>:"Add State(s) to Queue__jki_lib_state_machine.vi"("State(s) in Front (\"\")"=w311, "State(s) in (\"\")"=w315) -> ("States Out"=w314:string)  [unwired: 13 in]
          }
          frame "Macro: RC Exit" {
            n111 = Unbundle By Name(w319) -> ("RC Process Type"=w321)
            n112 = case shown="\"Client\"" w321 {
              tunnel: ["RC CM: Stop" ("State(s) in Front (\"\")") "RC: Close Connection\nProcess: SelfTerminate" ("State(s) in Front (\"\")") "RC: Close Connection\nProcess: SelfTerminate" ("State(s) in Front (\"\")")] -> w320
              frame "Connection Monitor", Default {
              }
              frame "Server" {
              }
              frame "Client" {
              }
            }
            n113 = call <vilib>:"Add State(s) to Queue__jki_lib_state_machine.vi"("State(s) in Front (\"\")"=w320, "State(s) in (\"\")"=w325) -> ("States Out"=w324:string)  [unwired: 13 in]
          }
          frame "Macro: Exit" {
            w339 = "UI: Front Panel State >> Close"  # UI: Front Panel State >> Close
            # "Exit Macro\n(This is called once, when the VI exits)"
            n114 = Unbundle By Name(w334) -> ("Core.Close Panel on Exit?"=w329)
            n115 = Select(t=w339, s=w329, f="") -> (s? t:f=w337:string)
            n116 = call <vilib>:"Add State(s) to Queue__jki_lib_state_machine.vi"("State(s) in Front (\"\")"="Macro: RC Exit\nData: Cleanup\nEvents: Unregister", "State(s) in (\"\")"="Process: Sync", "State(s) at Back (\"\")"="Exit") -> ("States Out"=w331:string)  [unwired: 12 in]
            n117 = call <vilib>:"Add State(s) to Queue__jki_lib_state_machine.vi"("State(s) in (\"\")"=w337, "State(s) at Back (\"\")"=w331) -> ("States Out"=w336:string)  [unwired: 13 in]
            n118 = call <vilib>:"Add State(s) to Queue__jki_lib_state_machine.vi"("State(s) in Front (\"\")"=w336, "State(s) in (\"\")"=w342) -> ("States Out"=w341:string)  [unwired: 13 in]
          }
          frame "---------- Process ----------" {
            # "Template Separator\n(You can make a copy of, or modify, this frame)"
            n119 = call <vilib>:"Add State(s) to Queue__jki_lib_state_machine.vi"("State(s) in (\"\")"=w347) -> ("States Out"=w346:string)  [unwired: 14 in]
          }
          frame "Process: Sync" {
            n120 = Unbundle By Name(w355) -> ("Self Reference"=w348)
            n121 = call <vilib>:"WaitOnProcessSync.vi"("error in (no error)"=w351, "SMO"=w348) -> ("error out"=w350:errorcluster, "Don't run?"=w354:bool)  [unwired: 7 in, 1 out]
            n122 = Select(t="Data: Cleanup\nEvents: Unregister\nExit", s=w354, f="") -> (s? t:f=w349:string)
            n123 = call <vilib>:"Add State(s) to Queue__jki_lib_state_machine.vi"("State(s) in Front (\"\")"=w349, "State(s) in (\"\")"=w358) -> ("States Out"=w357:string)  [unwired: 13 in]
          }
          frame "Process: SelfTerminate" {
            n124 = Unbundle By Name(w363) -> ("Self Reference"=w362)
            n125 = call <vilib>:"SelfTerminate.vi"("error in (no error)"=w360, "SMO in"=w362) -> ("error out"=w359:errorcluster, "SMO out"=w361:refnum<class "RemoteControl.lvclass">)  [unwired: 8 in]
            n126 = Bundle By Name(cluster=w363, "Self Reference"=w361) -> (w364:cluster{})
            n127 = call <vilib>:"Add State(s) to Queue__jki_lib_state_machine.vi"("State(s) in (\"\")"=w367) -> ("States Out"=w366:string)  [unwired: 14 in]
          }
          frame "---------- Events ----------" {
            # "Template Separator\n(You can make a copy of, or modify, this frame)"
            n128 = call <vilib>:"Add State(s) to Queue__jki_lib_state_machine.vi"("State(s) in (\"\")"=w372) -> ("States Out"=w371:string)  [unwired: 14 in]
          }
          frame "Events: Register" {
            w374 = refnum<user-event>[] [] items=["unknown", "Created", "Started", "Stopped"]  # Server State
            w373 = refnum<user-event>[] []  # Message From Server
            # "Expand to add\nmore events"
            n129 = Unbundle By Name(w385) -> ("Self Reference"=w376)
            n130 = call <vilib>:"GetProtectedEvents.vi"("SMO"=w376) -> ("error out"=w379:errorcluster, "SMO Protected Events"=w383:T10, "SMO out"=w375:refnum<class "RemoteControl.lvclass">)  [unwired: 8 in]
            n131 = call "RemoteControl.GetPrivateEvents.vi"("RemoteControl"=w375) -> ("error out"=w377:errorcluster, "RC Private Events"=w378:T11)  [unwired: 8 in, 1 out]
            n132 = register-events(w383, w378, w373, w374) -> (reference out=w384:refnum<event-registration>, error out=w380:errorcluster)  [unwired: 2 in]
            n133 = Merge Errors(w377, w382, w380, w379) -> (w381:errorcluster)
            n134 = call <vilib>:"Add State(s) to Queue__jki_lib_state_machine.vi"("State(s) in (\"\")"=w387) -> ("States Out"=w386:string)  [unwired: 14 in]
          }
          frame "Events: Unregister" {
            n135 = Unregister For Events(event registration refnum=w390, error in=w389) -> (error out=w388:errorcluster)
            n136 = call <vilib>:"Clear Errors.vi"("error in (no error)"=w388) -> ()  [unwired: 5 in, 2 out]
            n137 = call <vilib>:"Add State(s) to Queue__jki_lib_state_machine.vi"("State(s) in (\"\")"=w393) -> ("States Out"=w392:string)  [unwired: 14 in]
          }
          frame "---------- RC ----------" {
            # "Template Separator\n(You can make a copy of, or modify, this frame)"
            n138 = call <vilib>:"Add State(s) to Queue__jki_lib_state_machine.vi"("State(s) in (\"\")"=w398) -> ("States Out"=w397:string)  [unwired: 14 in]
          }
          frame "RC: Send Message to Owner" {
            # "Send a message to the instrument\nto be processed"
            # "If Connection Monitor: sends message from here to instrument\nIf Server: sends message from here to Connection Monitor"
            n139 = Unbundle By Name(w407) -> ("Self Reference"=w405, "Message"=w399)
            n140 = call "Time Message Events.vi"("error in (no error)"=w401, "Debug Mode"=w402, "Message in"=w399) -> ("error out"=w400:errorcluster, "Message out"=w403:T2)  [unwired: 6 in, 1 out]
            n141 = Bundle("Message out"=w403) -> (w404:cluster{"Message out":T2})  [unwired: 1 in]
            n142 = call "RemoteControl.SendMessageFromProcess.vi"("error in (no error)"=w400, "SendMessageFromProcess"=w404, "RemoteControl"=w405) -> ("error out"=w406:errorcluster)  [unwired: 7 in, 1 out]
            n143 = call <vilib>:"Add State(s) to Queue__jki_lib_state_machine.vi"("State(s) in (\"\")"=w410) -> ("States Out"=w409:string)  [unwired: 14 in]
          }
          frame "RC: Send Message to Server" {
            # "If Monitor: send message from here to server"
            n144 = Unbundle By Name(w421) -> ("Servers"=w413, "Server index"=w411, "Message"=w417)
            n145 = Index Array(array=w413, index=w411) -> (element=w412)
            n146 = call "Time Message Events.vi"("error in (no error)"=w415, "Debug Mode"=w418, "Message in"=w417) -> ("error out"=w414:errorcluster, "Message out"=w416:T2)  [unwired: 6 in, 1 out]
            n147 = Bundle("Message out"=w416) -> (w419:cluster{"Message out":T2})  [unwired: 1 in]
            n148 = call "RemoteControl.SendMessageToProcess.vi"("error in (no error)"=w414, "SendMessageToProcess"=w419, "RemoteControl"=w412) -> ("error out"=w420:errorcluster)  [unwired: 7 in, 1 out]
            n149 = call <vilib>:"Add State(s) to Queue__jki_lib_state_machine.vi"("State(s) in (\"\")"=w424) -> ("States Out"=w423:string)  [unwired: 14 in]
          }
          frame "RC: Read Message" {
            # "Read Message over, eg TCP"
            # "If command is empty do not Send Message"
            n150 = Unbundle By Name(w427) -> ("Message"=w430, "Self Reference"=w436)
            n151 = call-dynamic "Read Message.vi"("timeout in ms (100)"="timeout in ms (100)", "error in (no error)"=w437, "RemoteControl in"=w436) -> ("error out"=w429:errorcluster, "Data"=w432:variant, "Command"=w433:string, "Message ID"=w431:i32)  [unwired: 4 in, 1 out]
            n152 = case shown="Default" w433 {
              selector: w433 -> [w451 _]
              tunnel: ["RC: Send Message to Owner" ("State(s) in Front (\"\")") "" ("State(s) in Front (\"\")")] -> w435
              tunnel: w432 -> [w450 _]
              tunnel: w431 -> [w449 _]
              tunnel: w430 -> [w448 _]
              tunnel: w429 -> [w447 w453]
              tunnel: [w446 w453] -> w428
              tunnel: w427 -> [w445 w454]
              tunnel: [w444 w454] -> w426
              tunnel: w425 -> [w443 _]
              frame Default {
                n153 = Bundle By Name(cluster=w448, "Command"=w451, "Data"=w450, "Message ID"=w449) -> (w441:cluster{})
                "Message from Remote" <- w441
                n154 = call "Time Message Events.vi"("error in (no error)"=w447, "Debug Mode"=w443, "Message in"=w441) -> ("error out"=w446:errorcluster, "Message out"=w452:T2)  [unwired: 6 in, 1 out]
                n155 = Bundle By Name(cluster=w445, "Message"=w452) -> (w444:cluster{})
              }
              frame "" {
              }
            }
            n156 = call <vilib>:"Add State(s) to Queue__jki_lib_state_machine.vi"("State(s) in Front (\"\")"=w435, "State(s) in (\"\")"=w440) -> ("States Out"=w439:string)  [unwired: 13 in]
          }
          frame "RC: Write Message" {
            # "send Message over, eg. TCP"
            n157 = Unbundle By Name(w464) -> ("Self Reference"=w466, "Message"=w462)
            n158 = call "Time Message Events.vi"("error in (no error)"=w461, "Debug Mode"=w463, "Message in"=w462) -> ("error out"=w460:errorcluster, "Message out"=w459:T2)  [unwired: 6 in, 1 out]
            n159 = Unbundle By Name(w459) -> ("Command"=w458:string, "Data"=w457:variant, "Message ID"=w456:i32)
            n160 = call-dynamic "Send Message.vi"("Message ID"=w456, "error in (no error)"=w460, "Data"=w457, "Command"=w458, "RemoteControl in"=w466) -> ("error out"=w465:errorcluster)  [unwired: 5 in, 1 out]
            n161 = call <vilib>:"Add State(s) to Queue__jki_lib_state_machine.vi"("State(s) in (\"\")"=w469) -> ("States Out"=w468:string)  [unwired: 14 in]
          }
          frame "RC: Open Server Connection" {
            n162 = Unbundle By Name(w470) -> ("Self Reference"=w473)
            n163 = call-dynamic "Open Server Connection.vi"("error in (no error)"=w475, "RemoteControl in"=w473) -> ("error out"=w474:errorcluster, "RemoteControl out"=w472:refnum<class "RemoteControl.lvclass">)  [unwired: 8 in]
            n164 = Bundle By Name(cluster=w470, "Self Reference"=w472) -> (w471:cluster{})
            n165 = call <vilib>:"Add State(s) to Queue__jki_lib_state_machine.vi"("State(s) in (\"\")"=w478) -> ("States Out"=w477:string)  [unwired: 14 in]
          }
          frame "RC: Open Client Connection" {
            n166 = Unbundle By Name(w480) -> ("Self Reference"=w484)
            n167 = call-dynamic "Open Client Connection.vi"("error in (no error)"=w483, "RemoteControl in"=w484) -> ("error out"=w482:errorcluster, "RemoteControl out"=w481:refnum<class "RemoteControl.lvclass">)  [unwired: 8 in]
            n168 = Bundle By Name(cluster=w480, "Self Reference"=w481) -> (w479:cluster{})
            n169 = call <vilib>:"Add State(s) to Queue__jki_lib_state_machine.vi"("State(s) in (\"\")"=w487) -> ("States Out"=w486:string)  [unwired: 14 in]
          }
          frame "RC: Close Connection" {
            # "call this on error 66, etc (when connection\ndrops). check these in error handler"
            n170 = Unbundle By Name(w491) -> ("Self Reference"=w492)
            n171 = call-dynamic "Close Connection.vi"("error in (no error)"=w493, "RemoteControl in"=w492) -> ("error out"=w488:errorcluster, "RemoteControl out"=w489:refnum<class "RemoteControl.lvclass">)  [unwired: 8 in]
            n172 = Bundle By Name(cluster=w491, "Self Reference"=w489) -> (w490:cluster{})
            n173 = call <vilib>:"Add State(s) to Queue__jki_lib_state_machine.vi"("State(s) in (\"\")"=w496) -> ("States Out"=w495:string)  [unwired: 14 in]
          }
          frame "---------- RC CM ----------" {
            # "Template Separator\n(You can make a copy of, or modify, this frame)"
            n174 = call <vilib>:"Add State(s) to Queue__jki_lib_state_machine.vi"("State(s) in (\"\")"=w501) -> ("States Out"=w500:string)  [unwired: 14 in]
          }
          frame "RC CM: Start" {
            # "Start Connection Monitor\nStarts Listener"
            n175 = Unbundle By Name(w503) -> ("Self Reference"=w507, "Configure"=w506)
            n176 = call-dynamic "Connection Monitor - Start.vi"("error in (no error)"=w509, "Configure"=w506, "RemoteControl in"=w507) -> ("error out"=w508:errorcluster, "RemoteControl out"=w504:refnum<class "RemoteControl.lvclass">)  [unwired: 7 in]
            n177 = Bundle By Name(cluster=w503, "Self Reference"=w504) -> (w502:cluster{})
            n178 = call <vilib>:"Add State(s) to Queue__jki_lib_state_machine.vi"("State(s) in (\"\")"=w511) -> ("States Out"=w510:string)  [unwired: 14 in]
          }
          frame "RC CM: Monitor" {
            # "Here listen for new connections and then stop after timeout or if there's a new connection"
            n179 = Unbundle By Name(w515) -> ("Servers"=w516, "Self Reference"=w521)
            n180 = call-dynamic "Connection Monitor.vi"("error in (no error)"=w517, "RemoteControl in"=w521) -> ("error out"=w513:errorcluster, "Server out"=w512:refnum<class "RemoteControl.lvclass">)  [unwired: 7 in, 1 out]
            n181 = call <vilib>:"isStateMachineObject.vi"("error in (no error)"=w513, "SMO"=w512) -> ("error out"=w519:errorcluster, "is SMO?"=w523:bool, "SMO out"=w522:refnum<class "RemoteControl.lvclass">)  [unwired: 7 in]
            n182 = case shown="True" w523 {
              tunnel: w522 -> [_ w528]
              tunnel: w516 -> [_ w536]
              tunnel: ["" w534] -> w518
              tunnel: w515 -> [w526 w530]
              tunnel: [w526 w529] -> w514
              frame False {
                # "if no connections made do nothing"
              }
              frame True {
                n183 = Build Array (concatenate)(w536, w528) -> (w531:refnum<class "RemoteControl.lvclass">[])
                n184 = Array Size(array=w531) -> (size(s)=w533:i32)
                n185 = Decrement(x=w533) -> (x-1=w532:i32)
                n186 = Format Into String(format string="RC CM: Add Connection >> %d", w532) -> (resulting string=w534:string)  [unwired: 2 in, 1 out]
                n187 = Bundle By Name(cluster=w530, "Servers"=w531) -> (w529:cluster{})
              }
            }
            n188 = call <vilib>:"Add State(s) to Queue__jki_lib_state_machine.vi"("State(s) in Front (\"\")"=w518, "State(s) in (\"\")"=w525) -> ("States Out"=w524:string)  [unwired: 13 in]
          }
          frame "RC CM: Check Connections" {
            n189 = Unbundle By Name(w541) -> ("Servers"=w538)
            n190 = for {
              tunnel: w538 -> [w551]
              tunnel: w540 -> [w550]
              tunnel: [w546] -> w537 mode=indexing
              tunnel: [w545] -> w539
              n191 = call <vilib>:"isStateMachineObject.vi"("error in (no error)"=w550, "SMO"=w551) -> ("error out"=w547:errorcluster, "is SMO?"=w549:bool, "SMO out"=w548:refnum<class "RemoteControl.lvclass">)  [unwired: 7 in]
              n192 = case shown="True" w549 {
                tunnel: w548 -> [_ w557]
                tunnel: w547 -> [w553 w556]
                tunnel: [SMOState_--Enum."unknown" ("SMO State") w555] -> w546
                tunnel: [w553 w554] -> w545
                frame False {
                }
                frame True {
                  n193 = call <vilib>:"GetState.vi"("error in (no error)"=w556, "SMO"=w557) -> ("error out"=w554:errorcluster, "SMO State"=w555:T1)  [unwired: 7 in, 1 out]
                }
              }
            }
            "Servers" <- w537
            n194 = call <vilib>:"Add State(s) to Queue__jki_lib_state_machine.vi"("State(s) in (\"\")"=w544) -> ("States Out"=w543:string)  [unwired: 14 in]
          }
          frame "RC CM: Add Connection" {
            # "add new events here\nunwired events are\nunchanged"
            # "Here listen for new connections and then stop after timeout or if there's a new connection"
            n195 = Unbundle By Name(w571) -> ("Server Message"=w565, "Server State"=w566, "Servers"=w561)
            n196 = Decimal String To Number(string=w573) -> (number=w572:i32)  [unwired: 2 in, 1 out]
            n197 = Index Array(array=w561, index=w572) -> (element=w560)
            n198 = call "RemoteControl.GetPublicEvents.vi"("error in (no error)"=w564, "RemoteControl"=w560) -> ("error out"=w575:errorcluster, "RC Public Events"=w576:T12, "RemoteControl out"=w574:refnum<class "RemoteControl.lvclass">)  [unwired: 7 in]
            n199 = Unbundle(w576) -> ("SendMessageFromProcess"=w563:refnum<user-event>)
            n200 = call <vilib>:"GetPublicEvents.vi"("error in (no error)"=w575, "SMO"=w574) -> ("error out"=w577:errorcluster, "Public Events"=w567:T13)  [unwired: 7 in, 1 out]
            n201 = Build Array (concatenate)(w565, w563) -> (w559:refnum<user-event>[])
            n202 = Unbundle By Name(w567) -> ("State"=w562:refnum<user-event>)
            n203 = Build Array (concatenate)(w566, w562) -> (w558:refnum<user-event>[])
            n204 = register-events(reference=w569, w559, w558) -> (reference out=w568:refnum<event-registration>)  [unwired: 3 in, 1 out]
            n205 = Bundle By Name(cluster=w571, "Server Message"=w559, "Server State"=w558) -> (w570:cluster{})
            n206 = call <vilib>:"Add State(s) to Queue__jki_lib_state_machine.vi"("State(s) in (\"\")"=w579) -> ("States Out"=w578:string)  [unwired: 14 in]
          }
          frame "RC CM: Remove Connection" {
            # "Not sure yet if this is necessary"
            # "Start Connection Monitor\nStarts Listener"
            n207 = Unbundle By Name(w592) -> ("Server Message"=w585, "Server State"=w584, "Servers"=w583)
            n208 = Decimal String To Number(string=w590) -> (number=w586:i32)  [unwired: 2 in, 1 out]
            n209 = Delete From Array(array=w585, index=w586) -> (array with subset deleted=w582)  [unwired: 1 in, 1 out]
            n210 = Delete From Array(array=w584, index=w586) -> (array with subset deleted=w581)  [unwired: 1 in, 1 out]
            n211 = Delete From Array(array=w583, index=w586) -> (array with subset deleted=w580)  [unwired: 1 in, 1 out]
            n212 = register-events(reference=w588, w582, w581) -> (reference out=w587:refnum<event-registration>)  [unwired: 3 in, 1 out]
            n213 = Bundle By Name(cluster=w592, "Server Message"=w582, "Server State"=w581, "Servers"=w580) -> (w591:cluster{})
            n214 = call <vilib>:"Add State(s) to Queue__jki_lib_state_machine.vi"("State(s) in (\"\")"=w594) -> ("States Out"=w593:string)  [unwired: 14 in]
          }
          frame "RC CM: Stop" {
            n215 = Unbundle By Name(w598) -> ("Self Reference"=w597)
            n216 = call-dynamic "Connection Monitor - Stop.vi"("error in (no error)"=w596, "RemoteControl in"=w597) -> ("error out"=w595:errorcluster)  [unwired: 8 in, 1 out]
            n217 = call <vilib>:"Add State(s) to Queue__jki_lib_state_machine.vi"("State(s) in (\"\")"=w601) -> ("States Out"=w600:string)  [unwired: 14 in]
          }
        }
      }
    }
    frame Error {
    }
  }
  n218 = call-parent "Call Parent Method"("error in"=w8, "LevyLab"=w7) -> ("error out"=w5:errorcluster, "LevyLab out"=→"RemoteControl out":refnum<class "RemoteControl.lvclass">)  [unwired: 8 in]
  n219 = Merge Errors(w5, w4) -> (→"error out":errorcluster)
